vi "storeStateData.vi"(8 "error in (no error)":errorcluster, 9 "State Data":refnum<class "data.lvclass">, 10 "Current State":refnum<class "state.lvclass">, 11 "statemachine in":refnum<class "statemachine.lvclass">) -> (0 "error out":errorcluster, 2 "Data changed?":bool, 3 "statemachine out":refnum<class "statemachine.lvclass">)   [LabVIEW 2020, in "eos.lvlib" / "statemachine.lvclass"]
uses:
  statemachine.lvclass
  interfaces/data/data.lvclass
  interfaces/state/state.lvclass
  statemachine.lvclass/statemachine.ctl
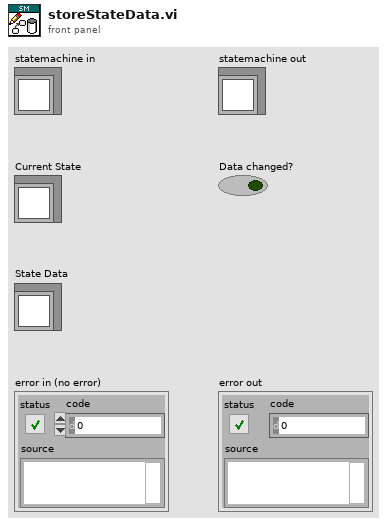
[diagram p1: front panel]
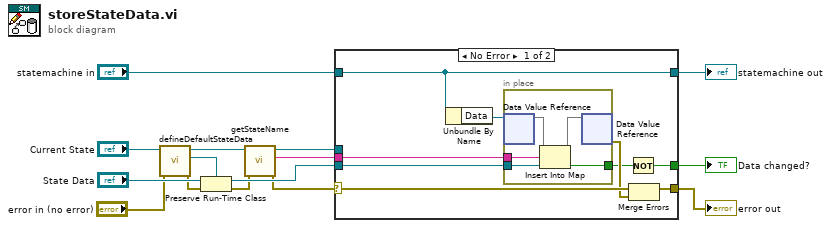
[diagram p0: block diagram]
diagram:
  n1 = call-dynamic "defineDefaultStateData.vi"("error in (no error)"="error in (no error)", "state in"="Current State") -> ("error out"=w5:errorcluster, "Default State Data"=w10:refnum<class "data.lvclass">, "state out"=w7:refnum<class "state.lvclass">)  [unwired: 7 in]
  n2 = Preserve Run-Time Class(object in="State Data", error in=w5, 2:w10) -> (object out=w12:refnum<class "data.lvclass">, error out=w4:errorcluster)
  n3 = call-dynamic "getStateName.vi"("error in (no error)"=w4, "state in"=w7) -> ("error out"=w3:errorcluster, "State Name"=w9:string, "state out"=w1:refnum<class "state.lvclass">)  [unwired: 7 in]
  n4 = case shown="No Error" w3 {
    selector: w3 -> [w22 w31]
    tunnel: w9 -> [w24 _]
    tunnel: w12 -> [w23 _]
    tunnel: [w20 w31] -> w13
    tunnel: [w17 _] -> w14
    tunnel: "statemachine in" -> [w16 w30]
    tunnel: [w16 w30] -> w15
    tunnel: w1 -> [_ _]
    frame No Error {
      n5 = Unbundle By Name(w16) -> ("Data"=w18:refnum<data-value>)
      n6 = in-place {
        in-place-border: w24 -> [w29]
        in-place-border: w23 -> [w28]
        in-place-border: [w27] -> w19
        n7 = in-place-dvr #1(w18) -> (w26:map{string, refnum<class "data.lvclass">})  [unwired: 1 out]
        n8 = Insert Into Map(map in=w26, key=w29, value=w28) -> (map out=w25:map{string, refnum<class "data.lvclass">}, value unchanged?=w27:bool)  [unwired: 1 out]
        n9 = in-place-dvr #1(w25) -> (w21:errorcluster)  [unwired: 1 out]
      }
      n10 = Not(x=w19) -> (.not. x?=w17:bool)
      n11 = Merge Errors(w22, w21) -> (w20:errorcluster)
    }
    frame Error {
    }
  }
  "statemachine out" <- w15
  "Data changed?" <- w14
  "error out" <- w13
